vi "BatteryReading.vi"(2 "SRV In":string) -> (1 "Battery ok?":bool, 4 "SRV Out":string="169.254.0.10")   [LabVIEW 2009]
panel:
  out "Reply":string
  # "This LabVIEW item is deprecated.\n\nIt is believed to be unused and will be removed in a future version of SRV."
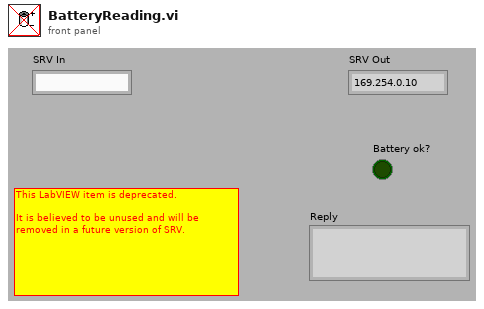
[diagram p1: front panel]
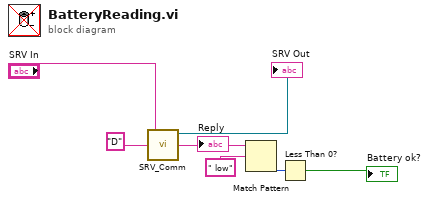
[diagram p0: block diagram]
diagram:
  n1 = call "SRV_Comm.vi"("Command Sent"="D", "SRV In"="SRV In") -> ("Reply"=w7:string, "SRV Out"=→"SRV Out":refnum<k5>)  [unwired: 1 in, 1 out]
  "Reply" <- w7
  n2 = Match Pattern(string=w7, regular expression=" low" ("Command Sent")) -> (offset past match=w1:i32)  [unwired: 1 in, 3 out]
  n3 = Less Than 0?(x=w1) -> (x < 0?=→"Battery ok?":bool)
